vi "DSF.Engine.Memory.Pointer.Channel Properties.Write.0D.vi"(8 "error in (no error)":errorcluster, 9 "value":T1 {"count" format="%d elements"; "size" format="%d bytes"; "offset" format="%d bytes"}, 10 "channel index":u64, 11 "Channel Properties Pointer in":refnum<class "DSF.Engine.Memory.Pointer.Channel Properties.lvclass">) -> (0 "error out":errorcluster, 3 "Channel Properties Pointer out":refnum<class "DSF.Engine.Memory.Pointer.Channel Properties.lvclass">)   [LabVIEW 2016, in "DSF.Engine.lvlib" / "DSF.Engine.Memory.Pointer.Channel Properties.lvclass"]
uses:
  DSF.Engine.Memory.Pointer.Channel Properties.lvclass
  C:/Git/SourceTree/DSF/Source/Engine/Classes/Pointer/DSF.Engine.Memory.Pointer.Array.lvclass
  C:/Git/SourceTree/DSF/Source/Submodules/Memory/Source/Classes/Pointer/Memory.Pointer.lvclass
  Shared/Typedefs/DSF.Shared.Typedefs.Channel Configuration.ctl
  Shared/Typedefs/DSF.Shared.Typedefs.Data Type.ctl
  DSF.Engine.Memory.Pointer.Array.lvclass/DSF.Engine.Memory.Pointer.Array.ctl
  Submodules/Memory/Source/Classes/Pointer/Memory.Pointer.lvclass/Memory.Pointer.ctl
  Submodules/Memory/Source/Classes/Pointer/Memory.Pointer.Errors.vi
  Submodules/Memory/Source/Classes/Pointer/Memory.Pointer.Errors.Out of Bounds.vi
  Submodules/Memory/Source/Classes/Pointer/Memory.Pointer.Get Size.vi
  Submodules/Memory/Source/Submodules/SEH/Source/VIs/Static Error Handling.Source Buffer.Write.String.vi
  Submodules/Memory/Source/Classes/Pointer/Memory.Pointer.Errors.Write Pointer Size.vi
  Submodules/Memory/Source/Classes/Pointer/Memory.Pointer.Errors.Create Error.vi
  Submodules/Memory/Source/Submodules/SEH/Source/VIs/Static Error Handling.Source Buffer.Write.Numeric.Scalar.Base10.vi
  Submodules/Memory/Source/Submodules/SEH/Source/VIs/Static Error Handling.Source Buffer.Write.Numeric.Scalar.Base10 (U64).vi
  Submodules/Memory/Source/Submodules/SEH/Source/VIs/Static Error Handling.Error Cluster Constant.vi
  Submodules/Memory/Source/Submodules/SEH/Source/VIs/Static Error Handling.Error Cluster Constant (256B).vi
  Submodules/Memory/Source/Submodules/SEH/Source/VIs/Static Error Handling.Parameters.Status.Set.vi
  Submodules/Memory/Source/Submodules/SEH/Source/VIs/Static Error Handling.Parameters.Code.Set.vi
  Submodules/Memory/Source/Submodules/SEH/Source/VIs/Static Error Handling.Parameters.VI Source.Set.vi
  Submodules/Memory/Source/Constants/Memory.Constants.vi
  Submodules/Memory/Source/Constants/Memory.Constants.Library Name.vi
  Submodules/Memory/Source/Classes/Pointer/Memory.Pointer.Errors.Get Info.vi
  DSF.Engine.Memory.Pointer.Array.lvclass
  Submodules/Memory/Source/Classes/Pointer/Memory.Pointer.lvclass
  DSF.Shared.lvlib
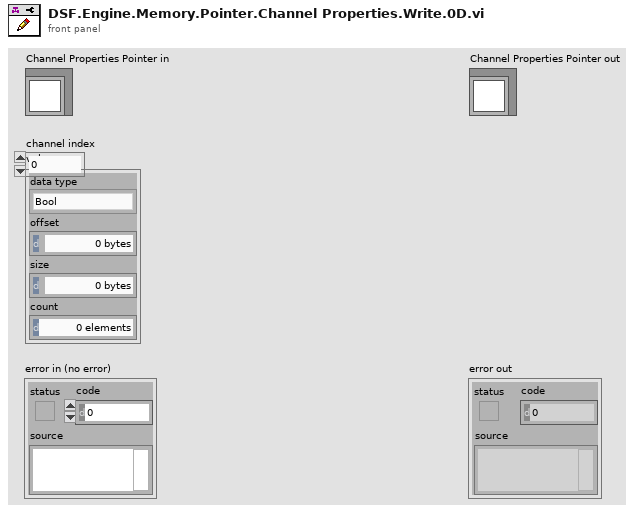
[diagram p1: front panel]
types:
  T1 = typedef "DSF.Shared.lvlib/DSF.Shared.Typedefs.Channel Configuration.ctl" = cluster{"data type":T2, "offset":u64, "size":u64, "count":u64}
  T2 = typedef "DSF.Shared.lvlib/DSF.Shared.Typedefs.Data Type.ctl" = enum8{"Bool", "SGL", "DBL", "I8", "I16", "I32", "I64", "U8", "U16", "U32", "U64"}
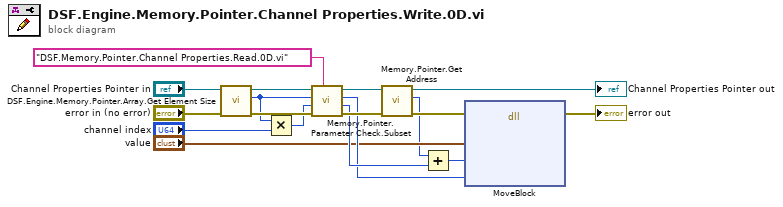
[diagram p0: block diagram]
diagram:
  n1 = call "DSF.Engine.Memory.Pointer.Array.Get Element Size.vi"("error in (no error)"="error in (no error)", "Array Pointer in"="Channel Properties Pointer in") -> ("error out"=w12:errorcluster, "element size"=w7:u64, "Array Pointer out"=w13:refnum<class "DSF.Engine.Memory.Pointer.Channel Properties.lvclass">)  [unwired: 7 in]
  n2 = Multiply(x=w7, y="channel index") -> (x*y=w8:u64)
  n3 = call "Memory.Pointer.Parameter Check.Subset.vi"("source vi name"="DSF.Memory.Pointer.Channel Properties.Read.0D.vi", "error in (no error)"=w12, "offset (0)"=w8, "length"=w7, "Pointer in"=w13) -> ("error out"=w10:errorcluster, "offset out"=w6:u64, "length"=w5:u64, "Pointer out"=w11:refnum<class "DSF.Engine.Memory.Pointer.Channel Properties.lvclass">)  [unwired: 3 in]
  n4 = call "Memory.Pointer.Get Address.vi"("error in (no error)"=w10, "Pointer in"=w11) -> ("error out"=w2:errorcluster, "address"=w1:u64, "Pointer out"=→"Channel Properties Pointer out":refnum<class "DSF.Engine.Memory.Pointer.Channel Properties.lvclass">)  [unwired: 7 in]
  n5 = Add(x=w1, y=w6) -> (x+y=w4:u64)
  n6 = dll-call lib="LabVIEW" fn="MoveBlock"(error in=w2, "src"="value", "dst"=w4, "size"=w5) -> (error out=→"error out":errorcluster)  [unwired: 6 in, 1 out]
